vi "SR_2000 Main.vi"(8 "Error In":errorcluster, 11 "Name":string) -> (0 "Error Out":errorcluster)   [LabVIEW 2019, in "SR_2000.lvlib"]
uses:
  SR_2000.lvlib
  Queue/Queue.lvlib
  Data Error Notifier/Data and Error Notifier.lvlib
panel:
  out "Port":u16
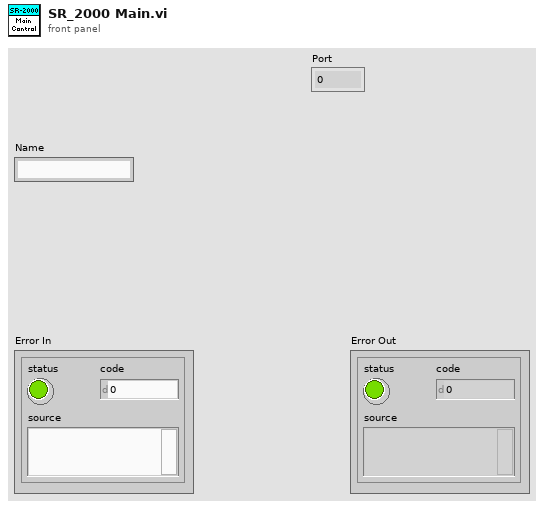
[diagram p1: front panel]
types:
  T1 = cluster{"NUMBER":u8, "Response data":string, "Read data":string}
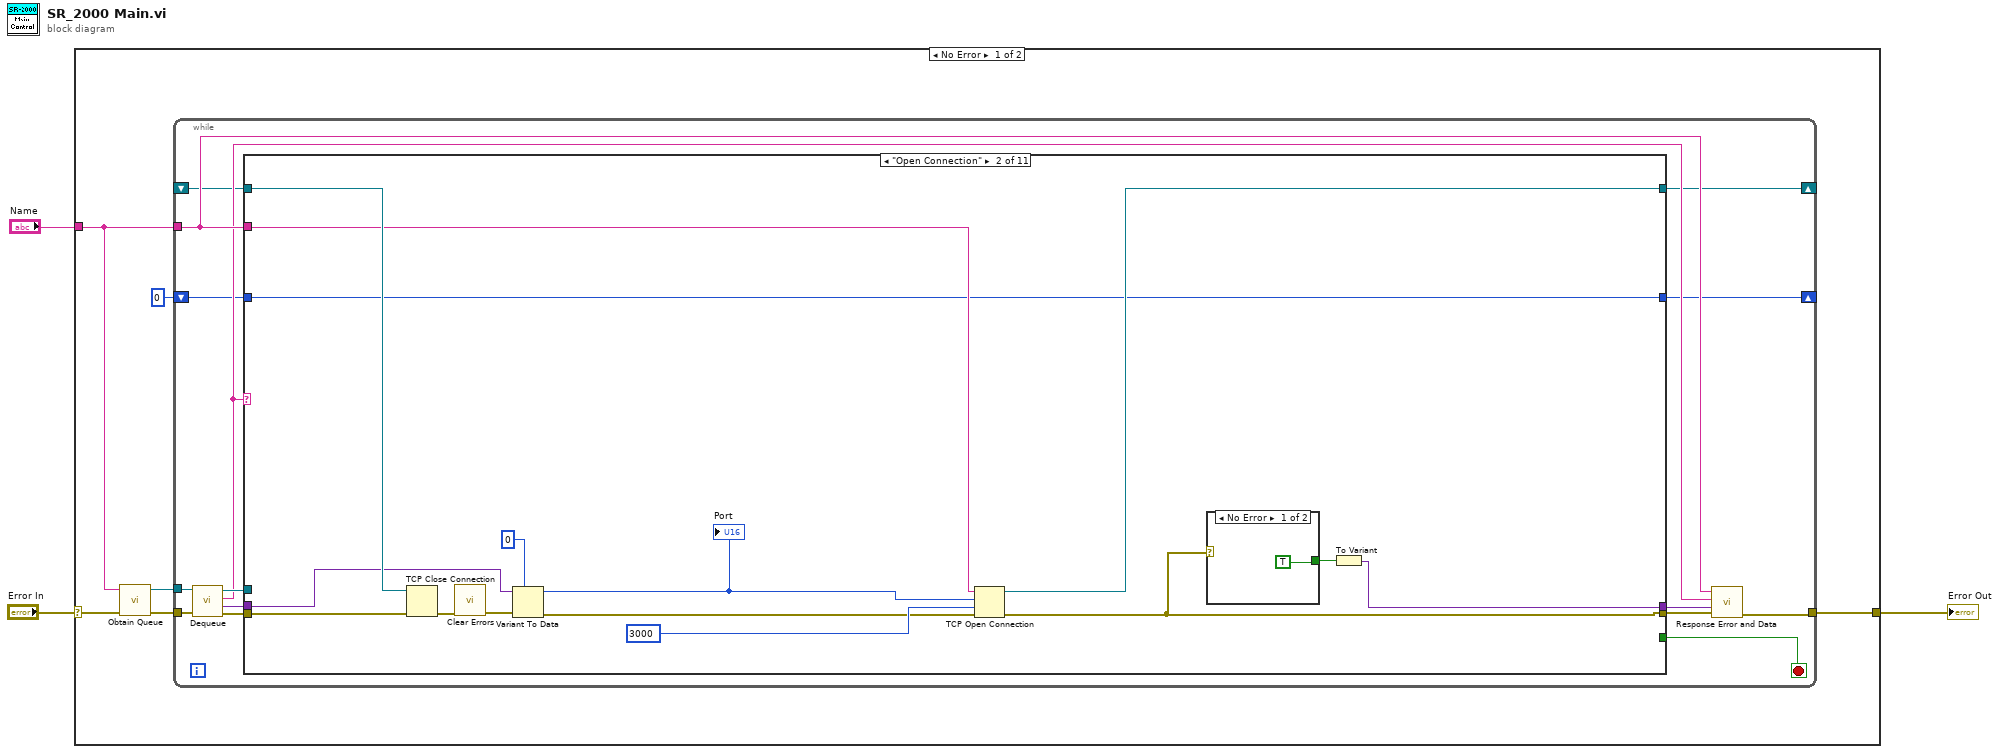
[diagram p0: block diagram]
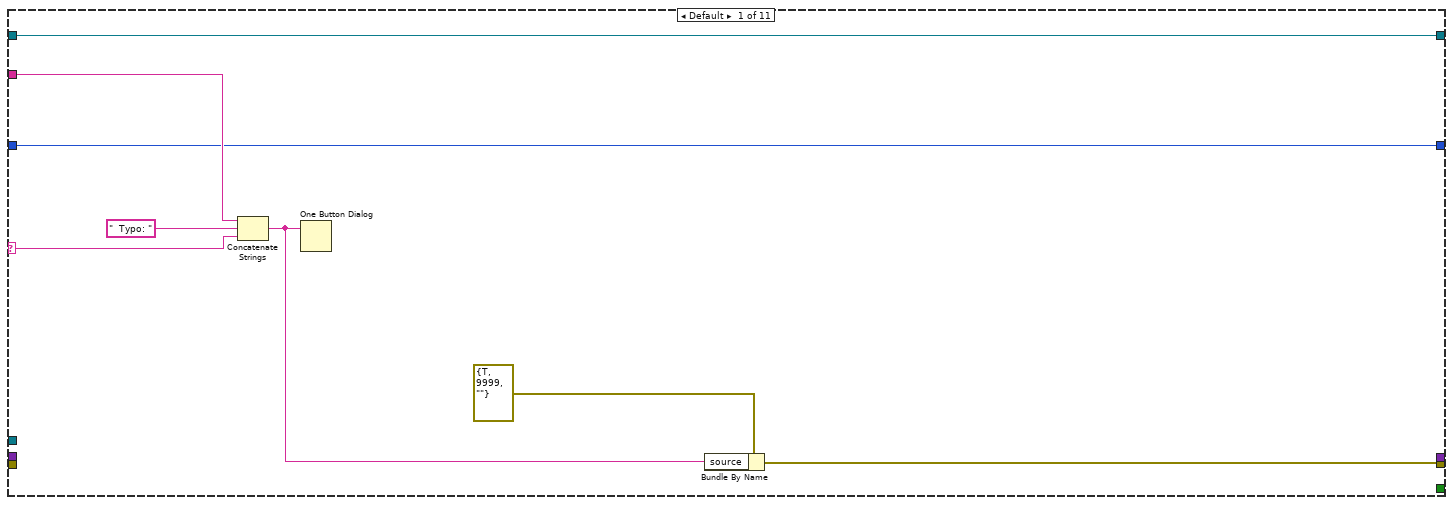
[diagram p2: hidden frame]
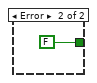
[diagram p3: hidden frame]
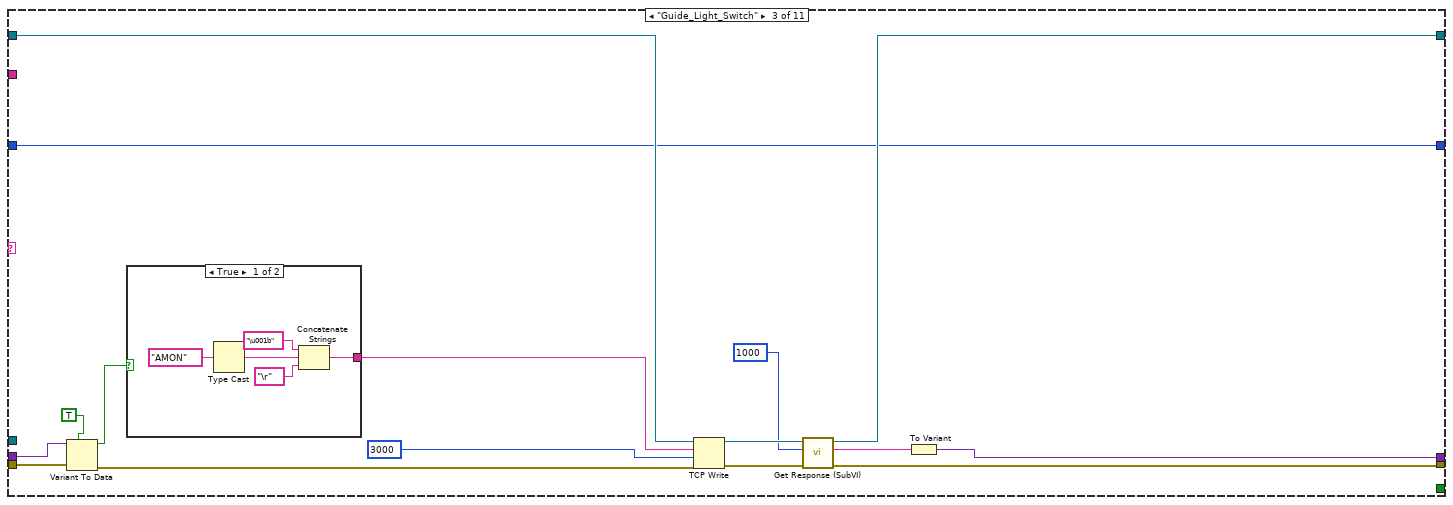
[diagram p4: hidden frame]
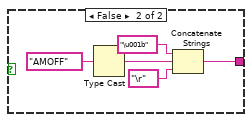
[diagram p5: hidden frame]
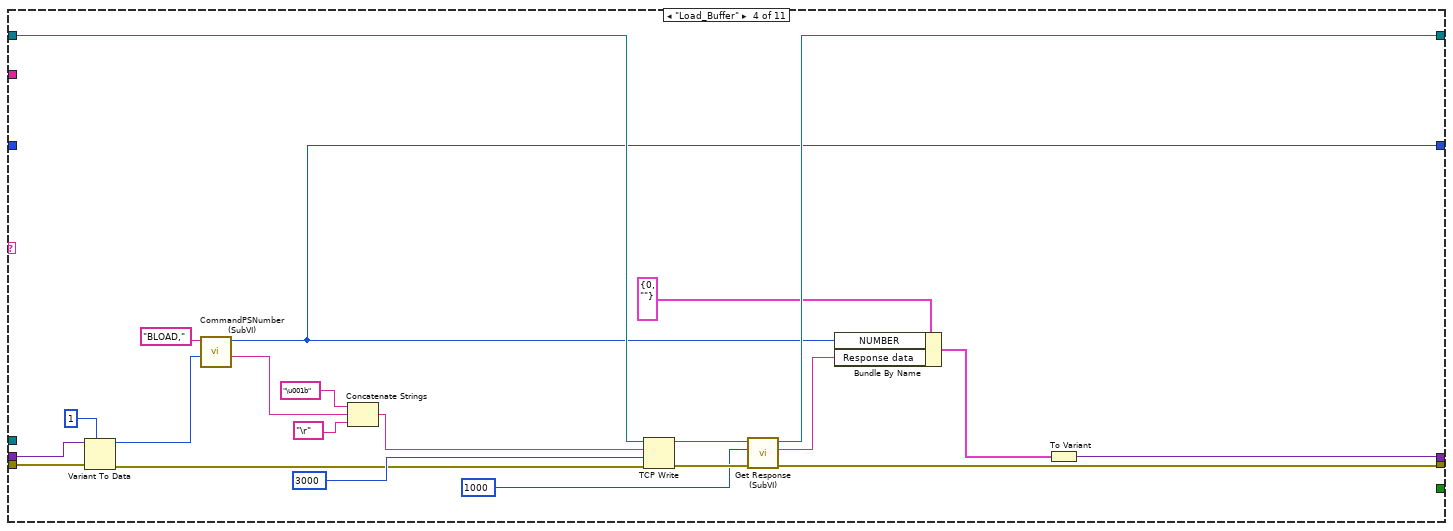
[diagram p6: hidden frame]
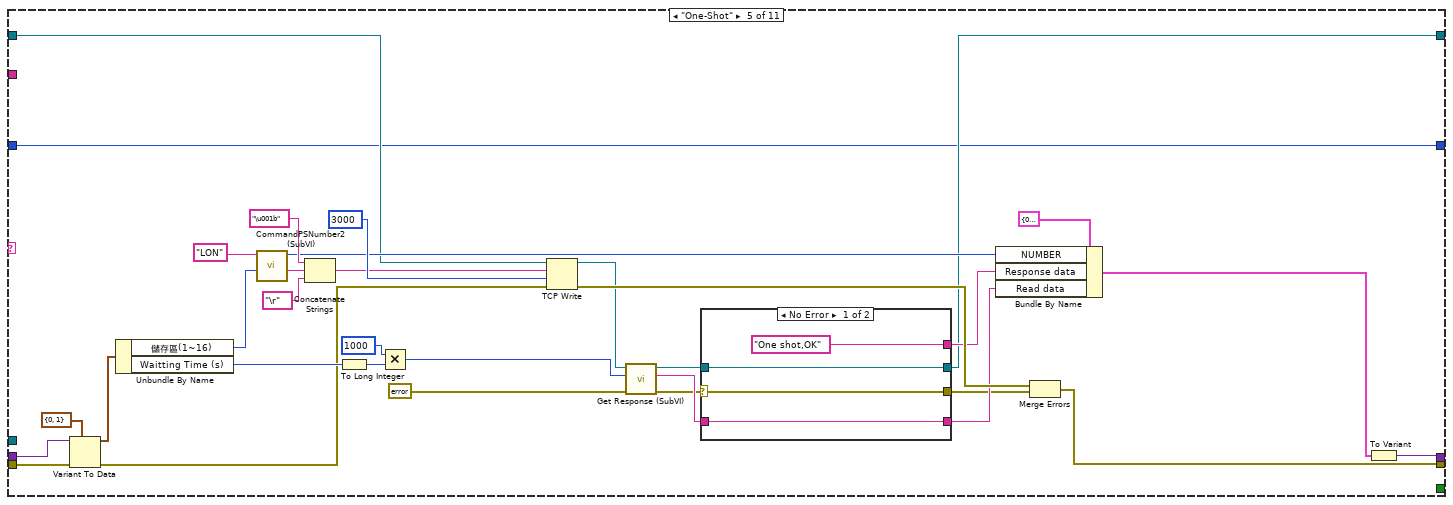
[diagram p7: hidden frame]
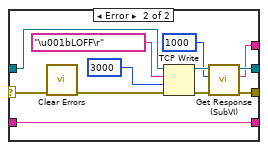
[diagram p8: hidden frame]
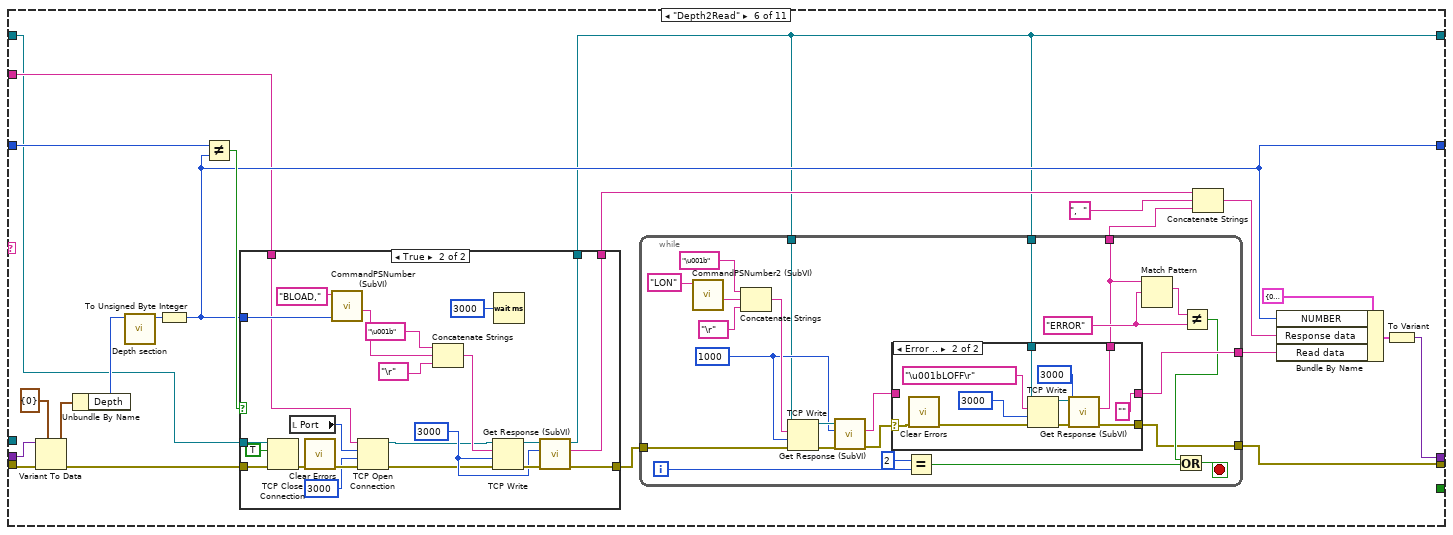
[diagram p9: hidden frame]
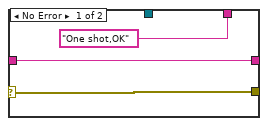
[diagram p10: hidden frame]
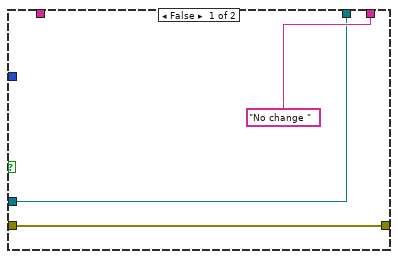
[diagram p11: hidden frame]
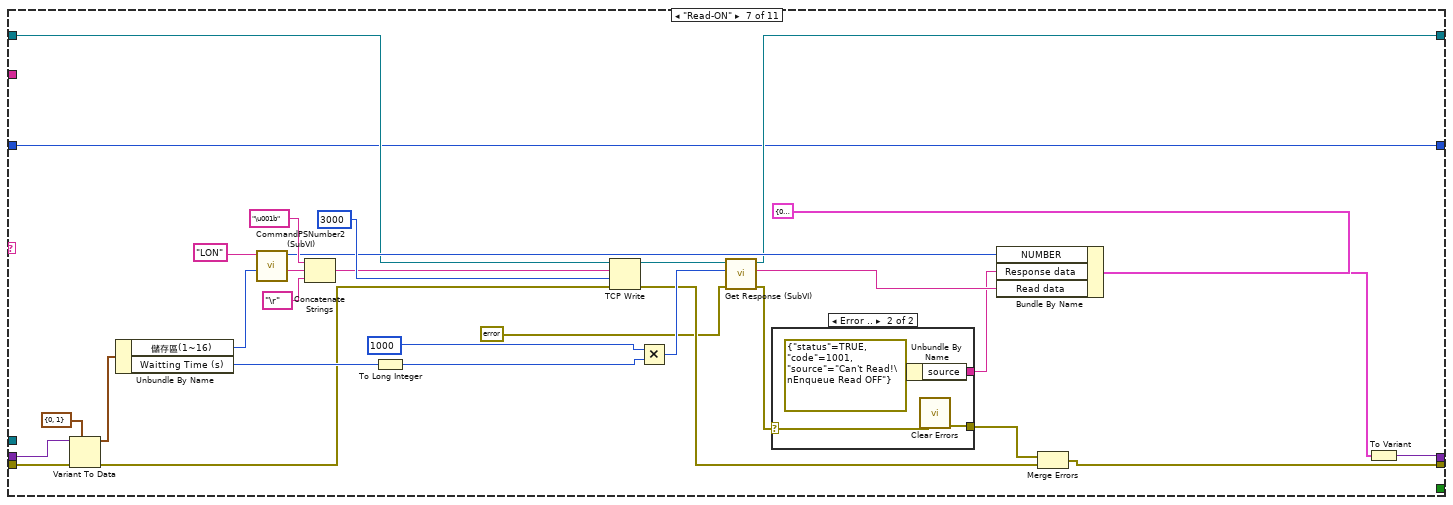
[diagram p12: hidden frame]
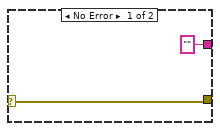
[diagram p13: hidden frame]
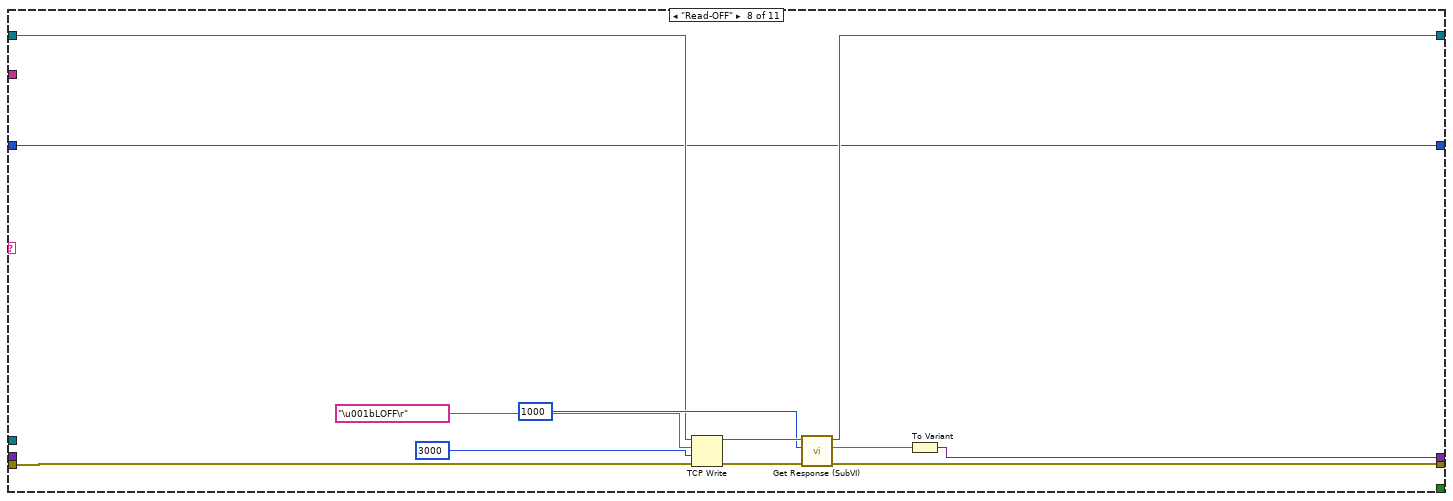
[diagram p14: hidden frame]
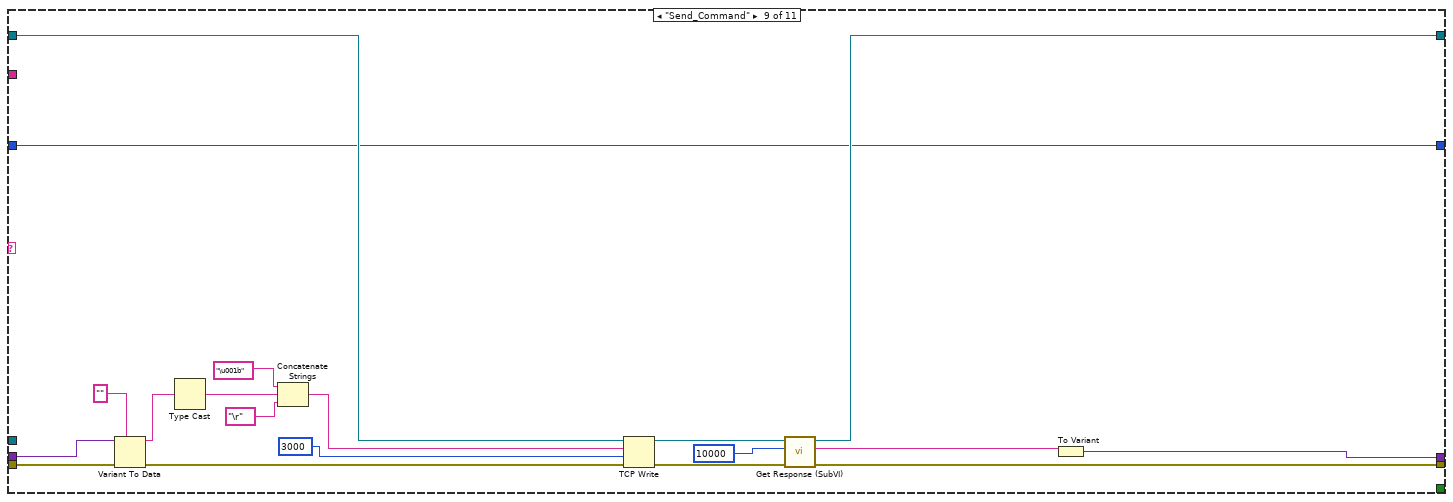
[diagram p15: hidden frame]
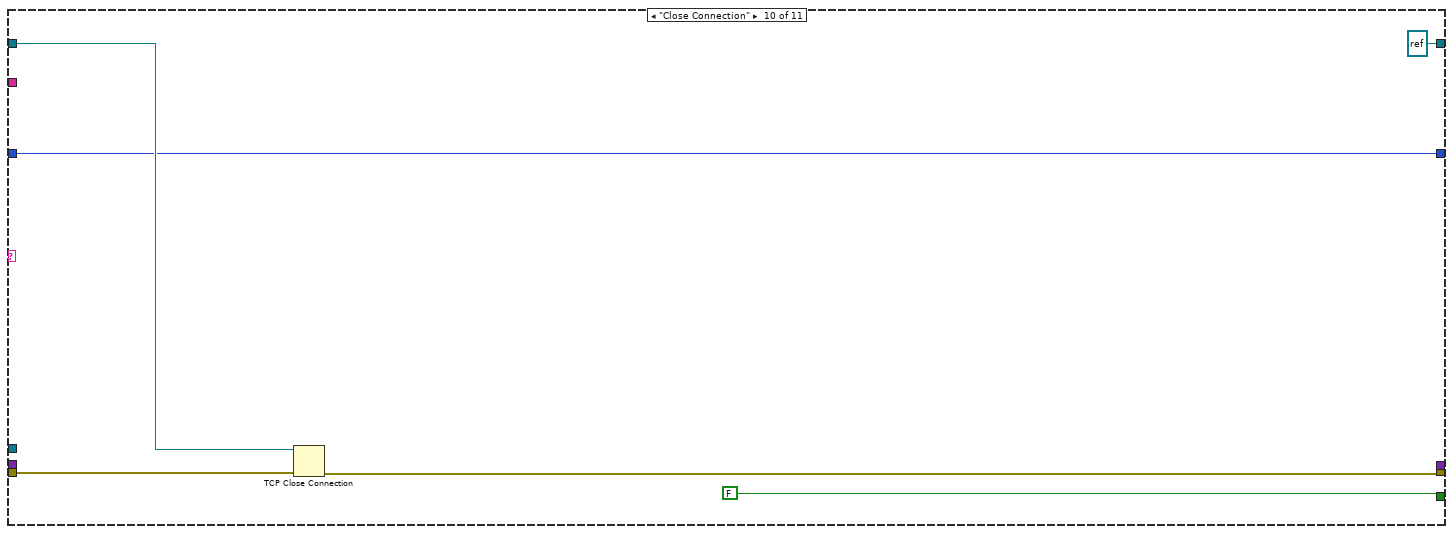
[diagram p16: hidden frame]
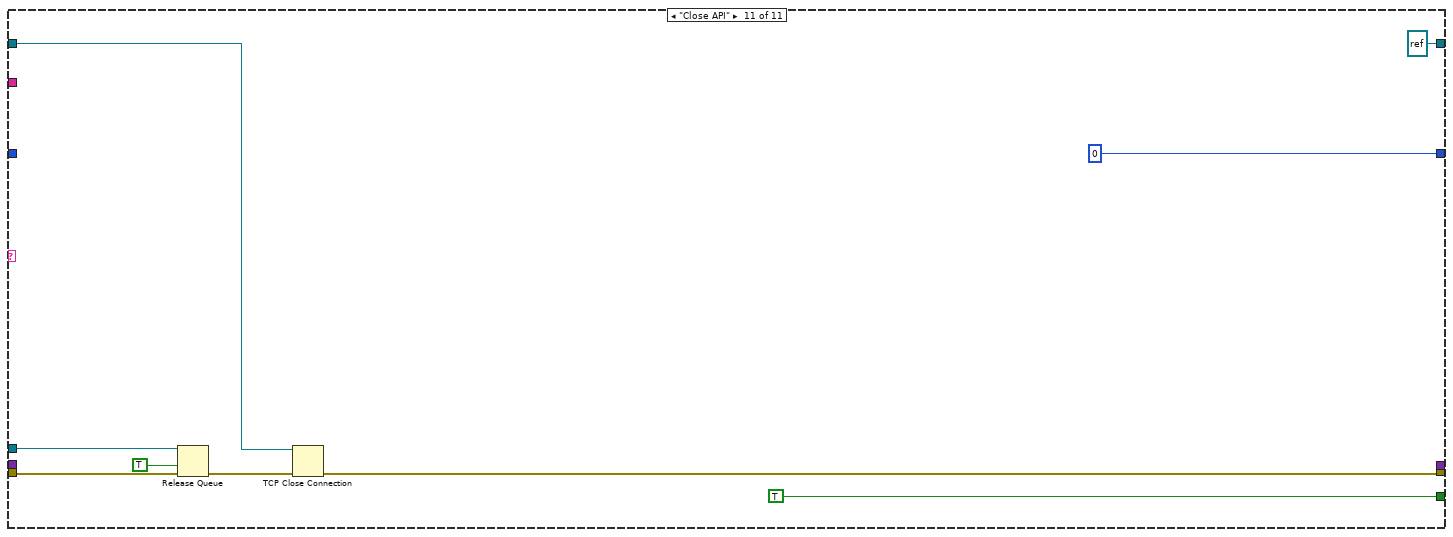
[diagram p17: hidden frame]
diagram:
  n1 = case shown="No Error" "Error In" {
    selector: "Error In" -> [w9 w316]
    tunnel: [w5 w316] -> w2
    tunnel: "Name" -> [w6 _]
    frame No Error {
      n2 = call "Obtain Queue.vi"("Error In"=w9, "Name"=w6) -> ("Error Out"=w8:errorcluster, "queue out"=w7:refnum<queue>)  [unwired: 8 in]
      n3 = while {
        tunnel: w8 -> [w24]
        tunnel: w7 -> [w22]
        tunnel: w6 -> [w17]
        tunnel: [w18] -> w5
        shift-right: [w14] -> _
        shift-left: _ -> [w15]
        shift-right: [w11] -> _
        shift-left: u8 0 ("NUMBER") -> [w10]
        stop <- w13 stop-if-true
        n4 = call "Dequeue.vi"("Error In"=w24, "queue in"=w22) -> ("Error Out"=w23:errorcluster, "Data"=w20:variant, "Message"=w16:string, "queue out"=w21:refnum<queue>)  [unwired: 6 in]
        n5 = case shown="\"Open Connection\"" w16 {
          selector: w16 -> [w30 _ _ _ _ _ _ _ _ _ _]
          tunnel: w23 -> [_ w47 w60 w88 w116 w165 w254 w276 w292 w306 w314]
          tunnel: w17 -> [w32 w40 _ _ _ w149 _ _ _ _ _]
          tunnel: w21 -> [_ _ _ _ _ _ _ _ _ _ w313]
          tunnel: [w27 w35 w53 w79 w109 w154 w238 w275 w283 w304 w310] -> w19
          tunnel: w20 -> [_ w43 w59 w87 w115 w164 w253 _ w291 _ _]
          tunnel: w15 -> [w25 w46 w54 w83 w103 w148 w236 w274 w286 w305 w311]
          tunnel: [w25 w39 w55 w82 w102 w147 w243 w273 w287 refnum<k5> refnum ("TCP Network Connection out") refnum<k5> refnum ("TCP Network Connection out")] -> w14
          tunnel: [_ _ _ _ _ _ _ _ _ FALSE TRUE] -> w13
          tunnel: [_ w33 w51 w78 w106 w156 w246 w271 w284 _ _] -> w12
          tunnel: [w26 w36 w50 w76 w98 w158 w233 w270 w282 w302 u8 0 ("NUMBER")] -> w11
          tunnel: w10 -> [w26 w36 w50 _ w98 w161 w233 w270 w282 w302 _]
          frame Default {
            n6 = Concatenate Strings(w32, "  Typo: " ("string"), w30) -> (w28:string)
            n7 = One Button Dialog(message=w28) -> ()  [unwired: 1 in, 1 out]
            n8 = Bundle By Name(cluster=errorcluster {"status"=TRUE, "code"=9999, "source"=""} ("Error In"), "source"=w28) -> (w27:errorcluster)
          }
          frame "Open Connection" {
            n9 = TCP Close Connection(connection ID=w46, error in (no error)=w47) -> (error out=w45:errorcluster)  [unwired: 1 in, 1 out]
            n10 = call <vilib>:"Clear Errors.vi"("error in (no error)"=w45) -> ("error out"=w44:errorcluster)  [unwired: 5 in, 1 out]
            n11 = Variant To Data(error in=w44, type=u16 0 ("Port"), Variant=w43) -> (data=w37:u16, error out=w41:errorcluster)
            "Port" <- w37
            n12 = TCP Open Connection(address=w40, remote port or service name=w37, timeout ms (60000)=3000, error in (no error)=w41) -> (connection ID=w39:refnum<k5>, error out=w35:errorcluster)  [unwired: 1 in]
            n13 = case shown="No Error" w35 {
              tunnel: [TRUE FALSE] -> w34
              frame No Error {
              }
              frame Error {
              }
            }
            n14 = To Variant(anything=w34) -> (Variant=w33:variant)
          }
          frame "Guide_Light_Switch" {
            n15 = Variant To Data(error in=w60, type=TRUE ("Test Switch"), Variant=w59) -> (data=w57:bool, error out=w56:errorcluster)
            n16 = case shown="True" w57 {
              tunnel: [w67 w72] -> w64
              frame True {
                n17 = Type Cast(x="AMON" ("data in")) -> (*(type *) &x=w69:string)  [unwired: 1 in]
                n18 = Concatenate Strings("\u001b" ("string"), w69, "\r") -> (w67:string)
              }
              frame False {
                n19 = Type Cast(x="AMOFF" ("data in")) -> (*(type *) &x=w74:string)  [unwired: 1 in]
                n20 = Concatenate Strings("\u001b" ("string"), w74, "\r") -> (w72:string)
              }
            }
            n21 = TCP Write(connection ID=w54, data in=w64, error in (no error)=w56, 9:3000 ("timeout ms (25000)")) -> (connection ID out=w62:refnum<k5>, error out=w63:errorcluster)  [unwired: 1 out]
            n22 = call "Get Response (SubVI).vi"("error in (no error)"=w63, "timeout ms (25000)"=1000, "TCP Network Connection in"=w62) -> ("error out"=w53:errorcluster, "Response data"=w52:string, "TCP Network Connection out"=w55:refnum<k5>)  [unwired: 6 in]
            n23 = To Variant(anything=w52) -> (Variant=w51:variant)
          }
          frame "Load_Buffer" {
            n24 = Variant To Data(error in=w88, type=u8 1 ("BUFFER NUMBER(1~8)"), Variant=w87) -> (data=w85:u8, error out=w84:errorcluster)
            n25 = call "CommandPSNumber (SubVI).vi"("BUFFER NUMBER(1~8)"=w85, "data in"="BLOAD,") -> ("COMMAND (Hex)"=w93:string, "NUMBER"=w76:u8)  [unwired: 8 in]
            n26 = Concatenate Strings("\u001b" ("string"), w93, "\r") -> (w95:string)
            n27 = TCP Write(connection ID=w83, data in=w95, error in (no error)=w84, 9:3000 ("timeout ms (25000)")) -> (connection ID out=w91:refnum<k5>, error out=w90:errorcluster)  [unwired: 1 out]
            n28 = call "Get Response (SubVI).vi"("error in (no error)"=w90, "timeout ms (25000)"=1000, "TCP Network Connection in"=w91) -> ("error out"=w79:errorcluster, "Response data"=w81:string, "TCP Network Connection out"=w82:refnum<k5>)  [unwired: 6 in]
            n29 = Bundle By Name(cluster=cluster{"NUMBER":u8, "Response data":string} {"NUMBER"=0, "Response data"=""}, "NUMBER"=w76, "Response data"=w81) -> (w77:cluster{"NUMBER":u8, "Response data":string})
            n30 = To Variant(anything=w77) -> (Variant=w78:variant)
          }
          frame "One-Shot" {
            n31 = Variant To Data(error in=w116, type=cluster{"Waitting Time (s)":u8, "儲存區(1~16)":u8} {"Waitting Time (s)"=0, "儲存區(1~16)"=1}, Variant=w115) -> (data=w114:cluster{"Waitting Time (s)":u8, "儲存區(1~16)":u8}, error out=w104:errorcluster)
            n32 = Unbundle By Name(w114) -> ("儲存區(1~16)"=w112:u8, "Waitting Time (s)"=w111:u8)
            n33 = call "CommandPSNumber2 (SubVI).vi"("Storage zone"=w112, "data in"="LON") -> ("COMMAND (Hex)"=w122:string, "NUMBER"=w108:u8)  [unwired: 8 in]
            n34 = Concatenate Strings("\u001b" ("string"), w122, "\r") -> (w118:string)
            n35 = To Long Integer(number=w111) -> (32bit integer=w126:i32)
            n36 = Multiply(x=1000, y=w126) -> (x*y=w125:i32)
            n37 = TCP Write(connection ID=w103, data in=w118, error in (no error)=w104, 9:3000 ("timeout ms (25000)")) -> (connection ID out=w123:refnum<k5>, error out=w130:errorcluster)  [unwired: 1 out]
            n38 = call "Get Response (SubVI).vi"("error in (no error)"=errorcluster {"status"=FALSE, "code"=0, "source"=""}, "timeout ms (25000)"=w125, "TCP Network Connection in"=w123) -> ("error out"=w127:errorcluster, "Response data"=w128:string, "TCP Network Connection out"=w129:refnum<k5>)  [unwired: 6 in]
            n39 = case shown="No Error" w127 {
              selector: w127 -> [w134 w143]
              tunnel: [w134 w137] -> w99
              tunnel: w128 -> [w132 w135]
              tunnel: ["One shot,OK" ("Response data") w138] -> w107
              tunnel: w129 -> [w133 w145]
              tunnel: [w133 w139] -> w102
              tunnel: [w132 w135] -> w100
              frame No Error {
              }
              frame Error {
                n40 = call <vilib>:"Clear Errors.vi"("error in (no error)"=w143) -> ("error out"=w142:errorcluster)  [unwired: 5 in, 1 out]
                n41 = TCP Write(connection ID=w145, data in="\u001bLOFF\r", error in (no error)=w142, 9:3000 ("timeout ms (25000)")) -> (connection ID out=w141:refnum<k5>, error out=w140:errorcluster)  [unwired: 1 out]
                n42 = call "Get Response (SubVI).vi"("error in (no error)"=w140, "timeout ms (25000)"=u32 1000, "TCP Network Connection in"=w141) -> ("error out"=w137:errorcluster, "Response data"=w138:string, "TCP Network Connection out"=w139:refnum<k5>)  [unwired: 6 in]
              }
            }
            n43 = Bundle By Name(cluster=T1 {"NUMBER"=0, "Response data"="", "Read data"=""}, "NUMBER"=w108, "Response data"=w107, "Read data"=w100) -> (w105:T1)
            n44 = Merge Errors(w130, w99) -> (w109:errorcluster)
            n45 = To Variant(anything=w105) -> (Variant=w106:variant)
          }
          frame "Depth2Read" {
            n46 = Variant To Data(error in=w165, type=cluster{"Depth":u16} {"Depth"=0}, Variant=w164) -> (data=w166:cluster{"Depth":u16}, error out=w160:errorcluster)
            n47 = Unbundle By Name(w166) -> ("Depth"=w162:u16)
            n48 = call "Depth section.vi"("深度資訊(mm)"=w162) -> ("Output section"=w169:u16)  [unwired: 10 in]
            n49 = To Unsigned Byte Integer(number=w169) -> (unsigned 8bit integer=w158:u8)
            n50 = Not Equal?(x=w161, y=w158) -> (x != y?=w168:bool)
            n51 = case shown="True" w168 {
              tunnel: w158 -> [_ w227]
              tunnel: [w209 w223] -> w167
              tunnel: w160 -> [w209 w218]
              tunnel: ["No change " ("Response data") w222] -> w153
              tunnel: w149 -> [_ w216]
              tunnel: w148 -> [w207 w217]
              tunnel: [w207 w212] -> w147
              frame False {
              }
              frame True {
                w224 = 3000 ("timeout ms (25000)")
                n52 = TCP Close Connection(connection ID=w217, abort (F)=TRUE, error in (no error)=w218) -> (error out=w221:errorcluster)  [unwired: 1 out]
                n53 = local read "Port"() -> (w215:u16)
                n54 = call <vilib>:"Clear Errors.vi"("error in (no error)"=w221) -> ("error out"=w220:errorcluster)  [unwired: 5 in, 1 out]
                n55 = call "CommandPSNumber (SubVI).vi"("BUFFER NUMBER(1~8)"=w227, "data in"="BLOAD,") -> ("COMMAND (Hex)"=w229:string)  [unwired: 8 in, 1 out]
                n56 = TCP Open Connection(address=w216, remote port or service name=w215, timeout ms (60000)=3000, error in (no error)=w220) -> (connection ID=w213:refnum<k5>, error out=w214:errorcluster)  [unwired: 1 in]
                n57 = Concatenate Strings("\u001b" ("string"), w229, "\r") -> (w231:string)
                n58 = TCP Write(connection ID=w213, data in=w231, error in (no error)=w214, 9:w224) -> (connection ID out=w225:refnum<k5>, error out=w226:errorcluster)  [unwired: 1 out]
                n59 = Wait (ms)(milliseconds to wait=u32 3000) -> ()  [unwired: 1 out]
                n60 = call "Get Response (SubVI).vi"("error in (no error)"=w226, "timeout ms (25000)"=w224, "TCP Network Connection in"=w225) -> ("error out"=w223:errorcluster, "Response data"=w222:string, "TCP Network Connection out"=w212:refnum<k5>)  [unwired: 6 in]
              }
            }
            n61 = while {
              tunnel: w167 -> [w184]
              tunnel: [w178] -> w155
              tunnel: [w173] -> w154
              tunnel: [w172] -> w151
              tunnel: w147 -> [w171]
              tunnel: w147 -> [w170]
              i -> [w192]
              stop <- w190 stop-if-true
              w174 = "ERROR" ("y")
              w182 = 1000 ("timeout ms (25000)")
              n62 = call "CommandPSNumber2 (SubVI).vi"("data in"="LON") -> ("COMMAND (Hex)"=w189:string)  [unwired: 9 in, 1 out]
              n63 = Concatenate Strings("\u001b" ("string"), w189, "\r") -> (w186:string)
              n64 = TCP Write(connection ID=w171, data in=w186, error in (no error)=w184, 9:w182) -> (connection ID out=w183:refnum<k5>, error out=w181:errorcluster)  [unwired: 1 out]
              n65 = call "Get Response (SubVI).vi"("error in (no error)"=w181, "timeout ms (25000)"=w182, "TCP Network Connection in"=w183) -> ("error out"=w180:errorcluster, "Response data"=w179:string)  [unwired: 6 in, 1 out]
              n66 = case shown="Error .." w180 {
                selector: w180 -> [w195 w205]
                tunnel: [w195 w200] -> w173
                tunnel: ["One shot,OK" ("Response data") w201] -> w172
                tunnel: w179 -> [w193 _]
                tunnel: [w193 "" ("Response data")] -> w178
                tunnel: w170 -> [_ w197]
                frame No Error {
                }
                frame Error {
                  n67 = call <vilib>:"Clear Errors.vi"("error in (no error)"=w205) -> ("error out"=w204:errorcluster)  [unwired: 5 in, 1 out]
                  n68 = TCP Write(connection ID=w197, data in="\u001bLOFF\r", error in (no error)=w204, 9:3000 ("timeout ms (25000)")) -> (connection ID out=w203:refnum<k5>, error out=w202:errorcluster)  [unwired: 1 out]
                  n69 = call "Get Response (SubVI).vi"("error in (no error)"=w202, "timeout ms (25000)"=3000, "TCP Network Connection in"=w203) -> ("error out"=w200:errorcluster, "Response data"=w201:string)  [unwired: 6 in, 1 out]
                }
              }
              n70 = Equal?(x=2, y=w192) -> (x = y?=w191:bool)
              n71 = Match Pattern(string=w172, regular expression=w174) -> (match substring=w175:string)  [unwired: 1 in, 3 out]
              n72 = Not Equal?(x=w175, y=w174) -> (x != y?=w176:bool)
              n73 = Or(x=w176, y=w191) -> (x .or. y?=w190:bool)
            }
            n74 = Concatenate Strings(w153, ",  " ("string"), w151) -> (w150:string)
            n75 = Bundle By Name(cluster=T1 {"NUMBER"=0, "Response data"="", "Read data"=""}, "NUMBER"=w158, "Response data"=w150, "Read data"=w155) -> (w157:T1)
            n76 = To Variant(anything=w157) -> (Variant=w156:variant)
          }
          frame "Read-ON" {
            n77 = Variant To Data(error in=w254, type=cluster{"Waitting Time (s)":u8, "儲存區(1~16)":u8} {"Waitting Time (s)"=0, "儲存區(1~16)"=1}, Variant=w253) -> (data=w252:cluster{"Waitting Time (s)":u8, "儲存區(1~16)":u8}, error out=w244:errorcluster)
            n78 = Unbundle By Name(w252) -> ("儲存區(1~16)"=w250:u8, "Waitting Time (s)"=w249:u8)
            n79 = call "CommandPSNumber2 (SubVI).vi"("Storage zone"=w250, "data in"="LON") -> ("COMMAND (Hex)"=w260:string, "NUMBER"=w247:u8)  [unwired: 8 in]
            n80 = Concatenate Strings("\u001b" ("string"), w260, "\r") -> (w256:string)
            n81 = To Long Integer(number=w249) -> (32bit integer=w263:i32)
            n82 = TCP Write(connection ID=w236, data in=w256, error in (no error)=w244, 9:3000 ("timeout ms (25000)")) -> (connection ID out=w235:refnum<k5>, error out=w240:errorcluster)  [unwired: 1 out]
            n83 = Multiply(x=1000, y=w263) -> (x*y=w262:i32)
            n84 = call "Get Response (SubVI).vi"("error in (no error)"=errorcluster {"status"=FALSE, "code"=0, "source"=""}, "timeout ms (25000)"=w262, "TCP Network Connection in"=w235) -> ("error out"=w241:errorcluster, "Response data"=w242:string, "TCP Network Connection out"=w243:refnum<k5>)  [unwired: 6 in]
            n85 = case shown="Error .." w241 {
              selector: w241 -> [w265 w268]
              tunnel: [w265 w269] -> w239
              tunnel: ["" ("source") w266] -> w234
              frame No Error {
              }
              frame Error {
                n86 = Unbundle By Name(errorcluster {"status"=TRUE, "code"=1001, "source"="Can't Read!\nEnqueue Read OFF"} ("Error In 2")) -> ("source"=w266:string)
                n87 = call <vilib>:"Clear Errors.vi"("error in (no error)"=w268) -> ("error out"=w269:errorcluster)  [unwired: 5 in, 1 out]
              }
            }
            n88 = Bundle By Name(cluster=T1 {"NUMBER"=0, "Response data"="", "Read data"=""}, "NUMBER"=w247, "Response data"=w234, "Read data"=w242) -> (w245:T1)
            n89 = Merge Errors(w239, w240) -> (w238:errorcluster)
            n90 = To Variant(anything=w245) -> (Variant=w246:variant)
          }
          frame "Read-OFF" {
            n91 = TCP Write(connection ID=w274, data in="\u001bLOFF\r", error in (no error)=w276, 9:3000 ("timeout ms (25000)")) -> (connection ID out=w279:refnum<k5>, error out=w278:errorcluster)  [unwired: 1 out]
            n92 = call "Get Response (SubVI).vi"("error in (no error)"=w278, "timeout ms (25000)"=1000, "TCP Network Connection in"=w279) -> ("error out"=w275:errorcluster, "Response data"=w272:string, "TCP Network Connection out"=w273:refnum<k5>)  [unwired: 6 in]
            n93 = To Variant(anything=w272) -> (Variant=w271:variant)
          }
          frame "Send_Command" {
            n94 = Variant To Data(error in=w292, type="", Variant=w291) -> (data=w289:string, error out=w288:errorcluster)
            n95 = Type Cast(x=w289) -> (*(type *) &x=w297:string)  [unwired: 1 in]
            n96 = Concatenate Strings("\u001b" ("string"), w297, "\r") -> (w299:string)
            n97 = TCP Write(connection ID=w286, data in=w299, error in (no error)=w288, 9:3000 ("timeout ms (25000)")) -> (connection ID out=w296:refnum<k5>, error out=w295:errorcluster)  [unwired: 1 out]
            n98 = call "Get Response (SubVI).vi"("error in (no error)"=w295, "timeout ms (25000)"=10000, "TCP Network Connection in"=w296) -> ("error out"=w283:errorcluster, "Response data"=w285:string, "TCP Network Connection out"=w287:refnum<k5>)  [unwired: 6 in]
            n99 = To Variant(anything=w285) -> (Variant=w284:variant)
          }
          frame "Close Connection" {
            n100 = TCP Close Connection(connection ID=w305, error in (no error)=w306) -> (error out=w304:errorcluster)  [unwired: 1 in, 1 out]
          }
          frame "Close API" {
            n101 = Release Queue(queue=w313, force destroy? (F)=TRUE, error in (no error)=w314) -> (error out=w312:errorcluster)  [unwired: 2 out]
            n102 = TCP Close Connection(connection ID=w311, error in (no error)=w312) -> (error out=w310:errorcluster)  [unwired: 1 in, 1 out]
          }
        }
        n103 = call "Response Error and Data.vi"("error in (no error)"=w19, "Data In"=w12, "Message"=w16, "Name"=w17) -> ("error out"=w18:errorcluster)  [unwired: 5 in, 2 out]
      }
    }
    frame Error {
    }
  }
  "Error Out" <- w2
